vi "clock.vi"() -> ()   [LabVIEW 2017]
panel:
  in  "Set Alarm":timestamp format="%<%X\n%x>T"
  out "date/time string 3":string
  out "date/time string 2":string
  out "date/time string":string
  out "current time":timestamp
  out "g 6":bool
  out "c 6":bool
  out "e 6":bool
  out "f 6":bool
  out "b 6":bool
  out "d 6":bool
  out "a 6":bool
  out "g 5":bool
  out "c 5":bool
  out "e 5":bool
  out "f 5":bool
  out "b 5":bool
  out "d 5":bool
  out "a 5":bool
  out "Boolean 4":bool
  out "Boolean 3":bool
  out "g 4":bool
  out "c 4":bool
  out "e 4":bool
  out "f 4":bool
  out "b 4":bool
  out "d 4":bool
  out "a 4":bool
  out "g 3":bool
  out "c 3":bool
  out "e 3":bool
  out "f 3":bool
  out "b 3":bool
  out "d 3":bool
  out "a 3":bool
  out "Boolean 2":bool
  out "Boolean":bool
  out "g 2":bool
  out "c 2":bool
  out "e 2":bool
  out "f 2":bool
  out "b 2":bool
  out "d 2":bool
  out "a 2":bool
  out "g":bool
  out "c":bool
  out "e":bool
  out "f":bool
  out "b":bool
  out "d":bool
  out "a":bool
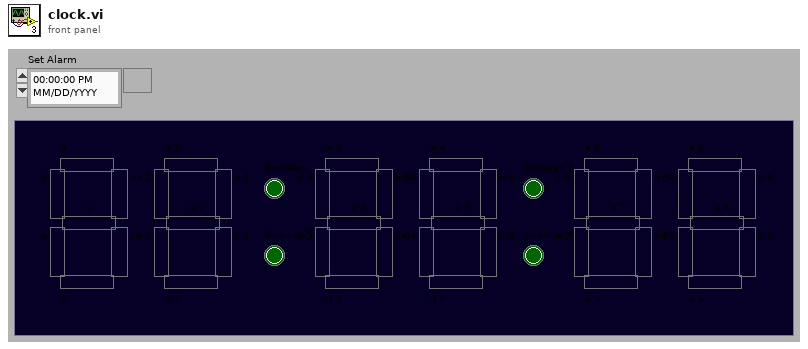
[diagram p1: front panel]
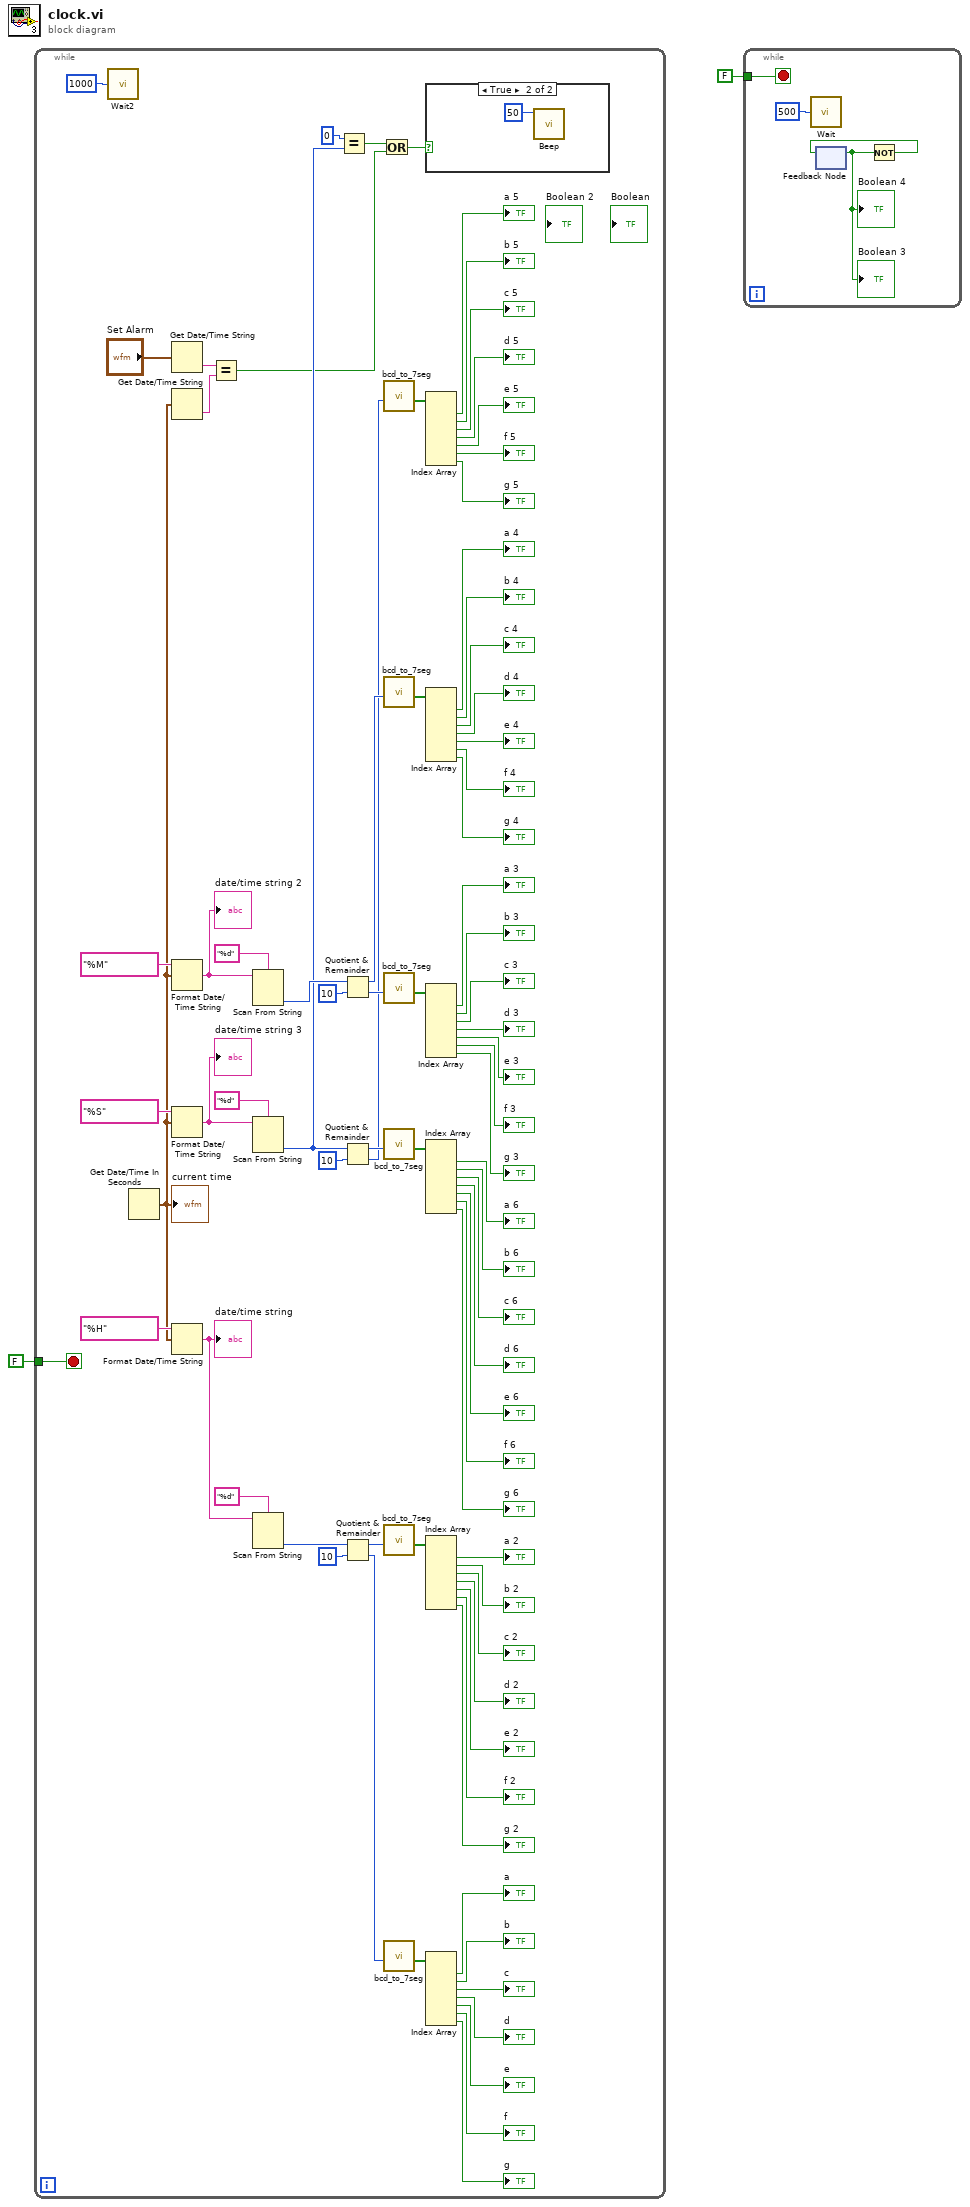
[diagram p0: block diagram]
diagram:
  n1 = while {
    tunnel: FALSE -> [w81]
    stop <- w81 stop-if-true
    n2 = call "Wait2"("Count(mSec)"=u16 1000) -> ()  [unwired: 1 out]
    n3 = Get Date/Time In Seconds() -> (seconds since 1Jan1904=w6:timestamp)
    "current time" <- w6
    n4 = Get Date/Time String(seconds (now)="Set Alarm") -> (time string=w3:string)  [unwired: 2 in, 1 out]
    n5 = Get Date/Time String(seconds (now)=w6) -> (time string=w4:string)  [unwired: 2 in, 1 out]
    n6 = Format Date/Time String(time format string (%c)="%M", seconds (now)=w6) -> (date/time string=w53:string)  [unwired: 1 in]
    "date/time string 2" <- w53
    n7 = Format Date/Time String(time format string (%c)="%S", seconds (now)=w6) -> (date/time string=w31:string)  [unwired: 1 in]
    "date/time string 3" <- w31
    n8 = Format Date/Time String(time format string (%c)="%H", seconds (now)=w6) -> (date/time string=w77:string)  [unwired: 1 in]
    "date/time string" <- w77
    n9 = Equal?(x=w3, y=w4) -> (x = y?=w7:bool)
    n10 = Scan From String(format string="%d", input string=w53) -> (output 1=w12:i32)  [unwired: 3 in, 3 out]
    n11 = Scan From String(format string="%d", input string=w31) -> (output 1=w10:i32)  [unwired: 3 in, 3 out]
    n12 = Scan From String(format string="%d", input string=w77) -> (output 1=w66:i32)  [unwired: 3 in, 3 out]
    n13 = Equal?(x=0, y=w10) -> (x = y?=w9:bool)
    n14 = Quotient & Remainder(x=w12, y=10) -> (x-y*floor(x/y)=w36:i32, floor(x/y)=w35:i32)
    n15 = Quotient & Remainder(x=w10, y=10) -> (x-y*floor(x/y)=w28:i32, floor(x/y)=w27:i32)
    n16 = Quotient & Remainder(x=w66, y=10) -> (x-y*floor(x/y)=w63:i32, floor(x/y)=w64:i32)
    n17 = Or(x=w9, y=w7) -> (x .or. y?=w8:bool)
    n18 = call "bcd_to_7seg.vi"("Number"=w27) -> ("7-Seg. Array"=w30:bool[])  [unwired: 10 in]
    n19 = call "bcd_to_7seg.vi"("Number"=w36) -> ("7-Seg. Array"=w52:bool[])  [unwired: 10 in]
    n20 = call "bcd_to_7seg.vi"("Number"=w35) -> ("7-Seg. Array"=w51:bool[])  [unwired: 10 in]
    n21 = call "bcd_to_7seg.vi"("Number"=w28) -> ("7-Seg. Array"=w29:bool[])  [unwired: 10 in]
    n22 = call "bcd_to_7seg.vi"("Number"=w63) -> ("7-Seg. Array"=w65:bool[])  [unwired: 10 in]
    n23 = call "bcd_to_7seg.vi"("Number"=w64) -> ("7-Seg. Array"=w67:bool[])  [unwired: 10 in]
    n24 = case shown="True" w8 {
      frame False {
      }
      frame True {
        n25 = call <vilib>:"Beep.vi"("frequency (Hz)"=50) -> ()  [unwired: 11 in]
      }
    }
    n26 = Index Array(array=w30) -> (element #1=→"a 5":bool, element #2=→"b 5":bool, element #3=→"c 5":bool, element #4=→"d 5":bool, element #5=→"e 5":bool, element #6=→"f 5":bool, element #7=→"g 5":bool)  [unwired: 7 in]
    n27 = Index Array(array=w52) -> (element #1=→"a 4":bool, element #2=→"b 4":bool, element #3=→"c 4":bool, element #4=→"d 4":bool, element #5=→"e 4":bool, element #6=→"f 4":bool, element #7=→"g 4":bool)  [unwired: 7 in]
    n28 = Index Array(array=w51) -> (element #1=→"a 3":bool, element #2=→"b 3":bool, element #3=→"c 3":bool, element #4=→"d 3":bool, element #5=→"e 3":bool, element #6=→"f 3":bool, element #7=→"g 3":bool)  [unwired: 7 in]
    n29 = Index Array(array=w29) -> (element #1=→"a 6":bool, element #2=→"b 6":bool, element #3=→"c 6":bool, element #4=→"d 6":bool, element #5=→"e 6":bool, element #6=→"f 6":bool, element #7=→"g 6":bool)  [unwired: 7 in]
    n30 = Index Array(array=w65) -> (element #1=→"a 2":bool, element #2=→"b 2":bool, element #3=→"c 2":bool, element #4=→"d 2":bool, element #5=→"e 2":bool, element #6=→"f 2":bool, element #7=→"g 2":bool)  [unwired: 7 in]
    n31 = Index Array(array=w67) -> (element #1=→"a":bool, element #2=→"b":bool, element #3=→"c":bool, element #4=→"d":bool, element #5=→"e":bool, element #6=→"f":bool, element #7=→"g":bool)  [unwired: 7 in]
  }
  n32 = while {
    tunnel: FALSE -> [w84]
    stop <- w84 stop-if-true
    n33 = call "Wait"("Count(mSec)"=500) -> ()  [unwired: 1 out]
    n34 = feedback #1() -> (w86:bool)  [unwired: 1 in]
    "Boolean 3" <- w86
    "Boolean 4" <- w86
    n35 = Not(x=w86) -> (.not. x?=w85:bool)
    n36 = feedback-in #1(w85) -> ()
  }
